vi "CANRead.vi"(11 "Double CAN in":T2) -> (0 "Data":T3[](array[typedef]) {"Data" format="%.0x"; "ArbitrationId" format="%.0x"; "Timestamp" format="%<%I:%M:%S%3u %p\n%m/%d/%Y>T"}, 3 "Double CAN out":T2)   [LabVIEW 2017]
uses:
  <vilib>/nican/nican.llb/CanFrameTimed.ctl
  <vilib>/nican/nican.llb/xobjhandle.ctl
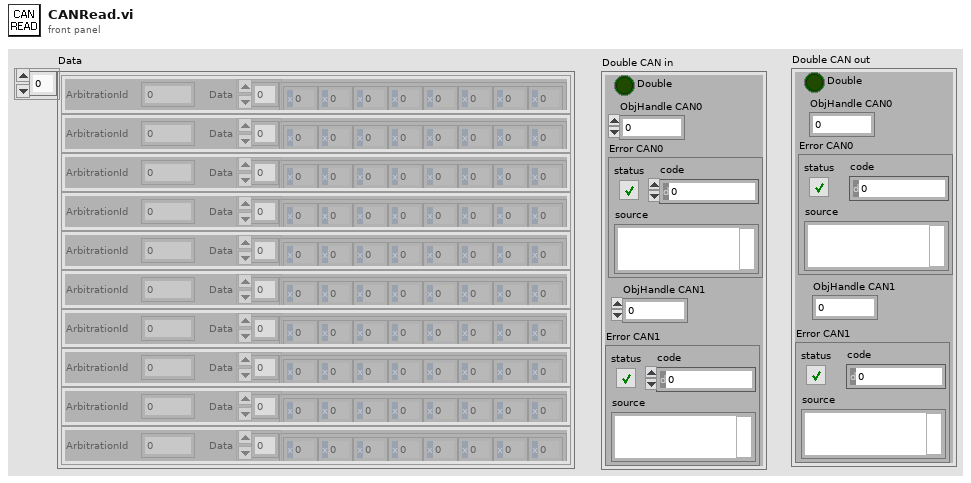
[diagram p1: front panel]
types:
  T1 = typedef "xobjhandle.ctl" = u32
  T2 = cluster{"ObjHandle CAN0":T1, "Error CAN0":errorcluster, "Error CAN1":errorcluster, "ObjHandle CAN1":T1, "Double":bool}
  T3 = typedef "CanFrameTimed.ctl" = cluster{"Timestamp":dbl, "ArbitrationId":u32, "IsRemote":u8, "DataLength":u8, "Data":u8[]}
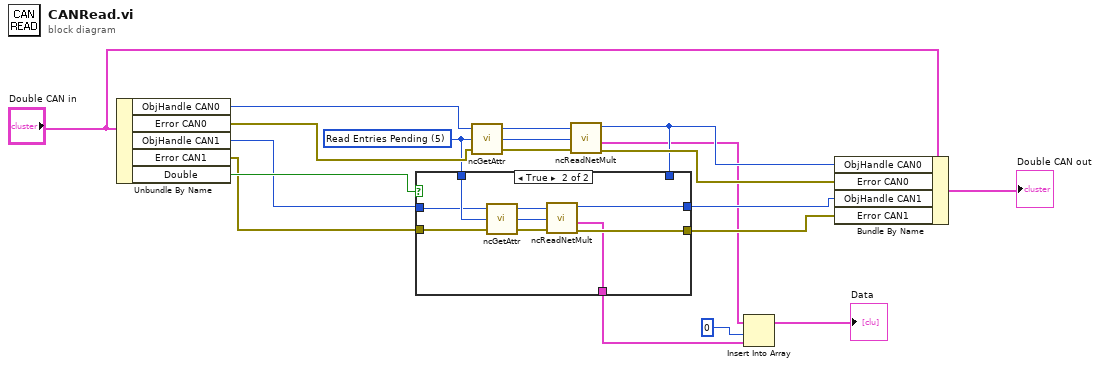
[diagram p0: block diagram]
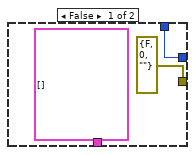
[diagram p2: hidden frame]
diagram:
  w11 = u32 5 items=["(reserved)", "Protocol Version", "Software Version", "Object State", "(reserved)", "Read Entries Pending", "Write Entries Pending", "ReadMult Size for Notification", "Listen Only?", "Self Reception?", "Transmit Error Counter", "Receive Error Counter", "Single Shot Transmit?", "Series 2 Filter Mode", "Series 2 Mask", "Series 2 Comparator", "Serial Number", "Form Factor", "Series", "Transceiver Type", "Interface Number", "Series 2 Error/Arb Capture", "Transceiver Mode", "Transceiver External Outputs", "Transceiver External Inputs", "Start Trigger Behavior", "Log Comm Warnings", "User RTSI Frame", "Transmit Mode", "Log Start Trigger?", "Timestamp Format", "Master Timebase Rate", "Virtual Bus Timing", "Write Entries Free", "Timeline Recovery", "Log Bus Errors", "Log Transceiver Faults", "Termination", "LIN Sleep", "LIN Checksum Type", "LIN Response Timeout", "LIN Enable DLC Check", "LIN Log Wakeup", "Baud Rate"] ("AttrId")
  n1 = Unbundle By Name("Double CAN in") -> ("ObjHandle CAN0"=w17:T1, "Error CAN0"=w16:errorcluster, "ObjHandle CAN1"=w10:T1, "Error CAN1"=w9:errorcluster, "Double"=w12:bool)
  n2 = call <vilib>:"ncGetAttr.vi"("Error in"=w16, "AttrId"=w11, "ObjHandle in"=w17) -> ("Error out"=w15:errorcluster, "AttrValue"=w19:u32, "ObjHandle out"=w18:T1)
  n3 = call <vilib>:"ncReadNetMult.vi"("ObjHandle in"=w18, "Requested Number of Frames"=w19, "Error in"=w15) -> ("ObjHandle out"=w5:T1, "Data"=w4:T3[], "Error out"=w6:errorcluster)  [unwired: 1 out]
  n4 = case shown="True" w12 {
    tunnel: w11 -> [_ w28]
    tunnel: w10 -> [_ w27]
    tunnel: w9 -> [_ w26]
    tunnel: [errorcluster {"status"=FALSE, "code"=0, "source"=""} ("Error out") w25] -> w8
    tunnel: [w22 w24] -> w7
    tunnel: w5 -> [w22 _]
    tunnel: [T3[] [] ("Data") w23] -> w3
    frame False {
    }
    frame True {
      n5 = call <vilib>:"ncGetAttr.vi"("Error in"=w26, "AttrId"=w28, "ObjHandle in"=w27) -> ("Error out"=w31:errorcluster, "AttrValue"=w29:u32, "ObjHandle out"=w30:T1)
      n6 = call <vilib>:"ncReadNetMult.vi"("ObjHandle in"=w30, "Requested Number of Frames"=w29, "Error in"=w31) -> ("ObjHandle out"=w24:T1, "Data"=w23:T3[], "Error out"=w25:errorcluster)  [unwired: 1 out]
    }
  }
  n7 = Insert Into Array(array=w4, index=0, new element=w3) -> (→"Data":T3[])
  n8 = Bundle By Name(cluster="Double CAN in", "ObjHandle CAN0"=w5, "Error CAN0"=w6, "ObjHandle CAN1"=w7, "Error CAN1"=w8) -> (→"Double CAN out":T2)
